vi "sub_erp42mini_sendata_conversion.vi"(11 "car_v":T1 {"speed_curr" format="%1_1g"; "Dir" scale=0.0..2.0; "Brake" scale=0.0..200.0; "Steer_set" scale=-2000.0..2000.0; "Acc_set" scale=0.0..10.0}) -> (3 "drive_v_strout":string)   [LabVIEW 2019]
panel:
  in  "Encoder_Reset_CMD":bool
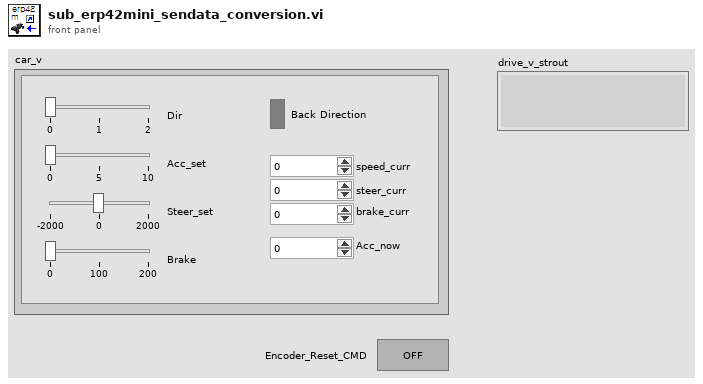
[diagram p1: front panel]
types:
  T1 = cluster{"Dir":u8, "Acc_set":u16, "Steer_set":i16, "Brake":i16, "Direction":bool, "speed_curr":dbl, "steer_curr":i16, "brake_curr":i16, "Acc_now":i16}
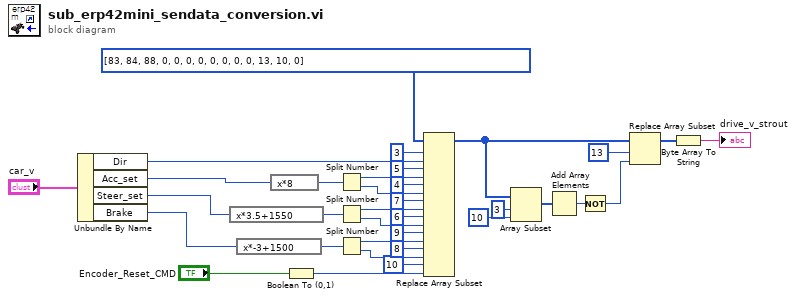
[diagram p0: block diagram]
diagram:
  n1 = Unbundle By Name("car_v") -> ("Dir"=w6:u8, "Acc_set"=w5:u16, "Steer_set"=w4:i16, "Brake"=w3:i16)
  n2 = expression code="x*3.5+1550"(w4) -> (w9:i16)
  n3 = expression code="x*-3+1500"(w3) -> (w8:i16)
  n4 = expression code="x*8"(w5) -> (w10:u16)
  n5 = Boolean To (0,1)(Boolean="Encoder_Reset_CMD") -> (0, 1=w7:i16)
  n6 = Split Number(x=w10) -> (hi(x)=w29:u8, lo(x)=w30:u8)
  n7 = Split Number(x=w9) -> (hi(x)=w31:u8, lo(x)=w32:u8)
  n8 = Split Number(x=w8) -> (hi(x)=w33:u8, lo(x)=w34:u8)
  n9 = Replace Array Subset(array=u8[] [83, 84, 88, 0, 0, 0, 0, 0, 0, 0, 0, 13, 10, 0] ("unsigned byte array"), new element #1=w6, index #1=3, new element #2=w29, index #2=5, new element #3=w30, index #3=4, new element #4=w31, index #4=7, new element #5=w32, index #5=6, new element #6=w33, index #6=9, new element #7=w34, index #7=8, new element #8=w7, index #8=10) -> (w11:u8[])
  n10 = Array Subset(array=w11, index=3, length=10) -> (w22:u8[])
  n11 = Add Array Elements(numeric array=w22) -> (sum=w23:u8)
  n12 = Not(x=w23) -> (.not. x?=w25:u8)
  n13 = Replace Array Subset(array=w11, new element=w25, index=13) -> (w27:u8[])
  n14 = Byte Array To String(unsigned byte array=w27) -> (string=→"drive_v_strout":string)
